vi "OCP.vi"(3 "Data In":dbl[][](array[numeric]), 4 "Timing":T7={"Resolution (ms)"=0.0, "index"=0, "Duty cycle array size"=0, "Pre-scan rest (ms)"=2000}, 9 "Arduino In":cluster{"error in":errorcluster, "LINX  in":T1}) -> (0 "Data Out":dbl[][](array[numeric]), 1 "Aquisition":T8, 2 "Stop condition":bool, 6 "Arduino Out":cluster{"error out":errorcluster, "LINX out":T1})   [LabVIEW 2022 SP3]
uses:
  <vilib>/MakerHub/LINX/Private/Type Defs/LINX Ref.ctl
  <vilib>/MakerHub/LINX/Private/Type Defs/Platform.ctl
  <vilib>/MakerHub/LINX/Private/Type Defs/Interface.ctl
  <vilib>/MakerHub/LINX/Private/Device/Type Defs/LINX Device Config.ctl
  <vilib>/MakerHub/LINX/Private/Device/Type Defs/TCP Config.ctl
  <vilib>/MakerHub/LINX/Private/Device/Type Defs/Channels.ctl
  <vilib>/MakerHub/LINX/Public/Peripherals/Analog/Analog Read 1 Chan.vi
  <vilib>/MakerHub/LINX/Public/Peripherals/Analog/Analog Read N Chans.vi
  <vilib>/MakerHub/LINX/Private/Local IO/LinxAnalogRead.vi
  <vilib>/MakerHub/LINX/Public/Utilities/Check Channel.vi
  <vilib>/MakerHub/LINX/Private/Utilties/Generate Error.vi
  <vilib>/MakerHub/LINX/LMH-LINX.lvlib
  <vilib>/MakerHub/LINX/Private/Device/Device.lvlib
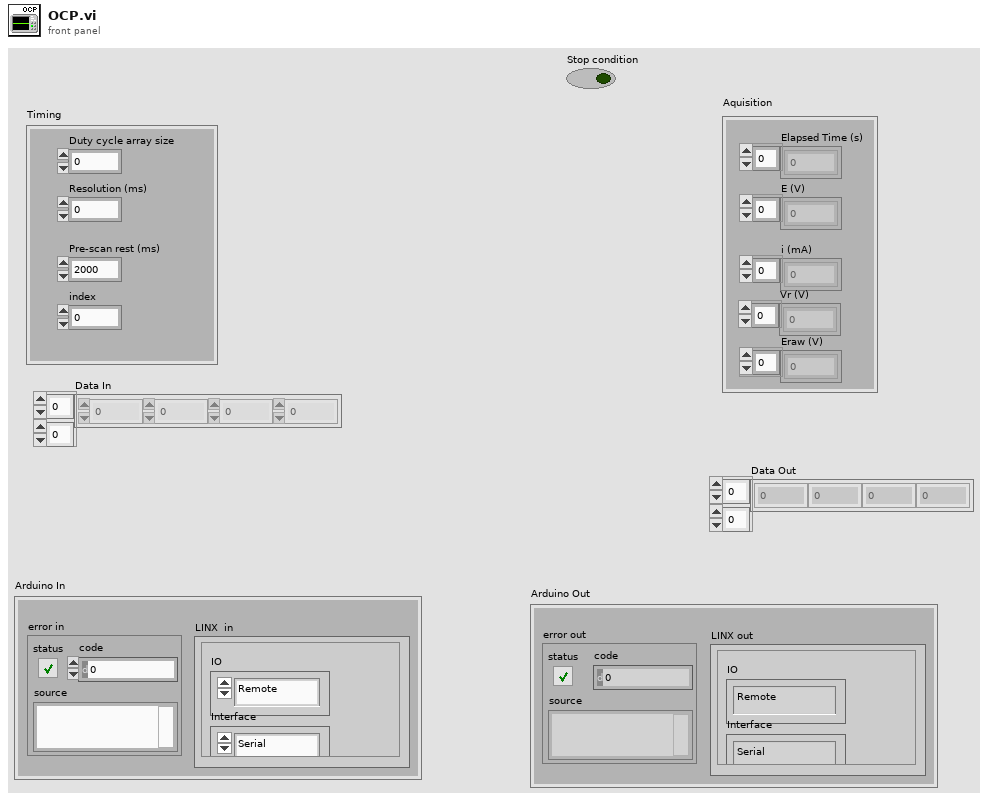
[diagram p1: front panel]
types:
  T1 = typedef "LMH-LINX.lvlib/LINX Ref.ctl" = cluster{"IO":T2, "Interface":T3, "LINX Device Config":T4}
  T2 = typedef "LMH-LINX.lvlib/Platform.ctl" = enum16{"Remote", "Local"}
  T3 = typedef "LMH-LINX.lvlib/Interface.ctl" = enum16{"Serial", "TCP"}
  T4 = typedef "LMH-LINX.lvlib/Device.lvlib/LINX Device Config.ctl" = cluster{"Interface":T3, "COM Port":refnum<visa-resource-name>, "TCP Configuration":T5, "Device Family":u8, "Device ID":u8, "Device Name":string, "TCP Ref":refnum<k5>, "Channels":T6}
  T5 = typedef "LMH-LINX.lvlib/Device.lvlib/TCP Config.ctl" = cluster{"IP Address":string, "Port":u16}
  T6 = typedef "LMH-LINX.lvlib/Channels.ctl" = cluster{"DI":u8[], "DO":u8[], "AI":u8[], "AO":u8[], "PWM":u8[], "QE":u8[], "UART":u8[], "I2C 2":u8[], "SPI":u8[], "CAN":u8[], "Servo":u8[], "AI Ref (V)":dbl, "AI Resolution (Bits)":u8, "AO Ref (V)":dbl, "AO Resolution (Bits)":u8}
  T7 = cluster{"Resolution (ms)":dbl, "index":i32, "Duty cycle array size":i32, "Pre-scan rest (ms)":u32}
  T8 = cluster{"Elapsed Time (s)":dbl[], "E (V)":dbl[], "i (mA)":dbl[], "Vr (V)":dbl[], "Eraw (V)":dbl[]}
  T9 = cluster{"Error Out":errorcluster, "LINX Resource":T1}
  T10 = cluster{dbl[], dbl[], "subarray":dbl[], "subarray":dbl[], "subarray":dbl[]}
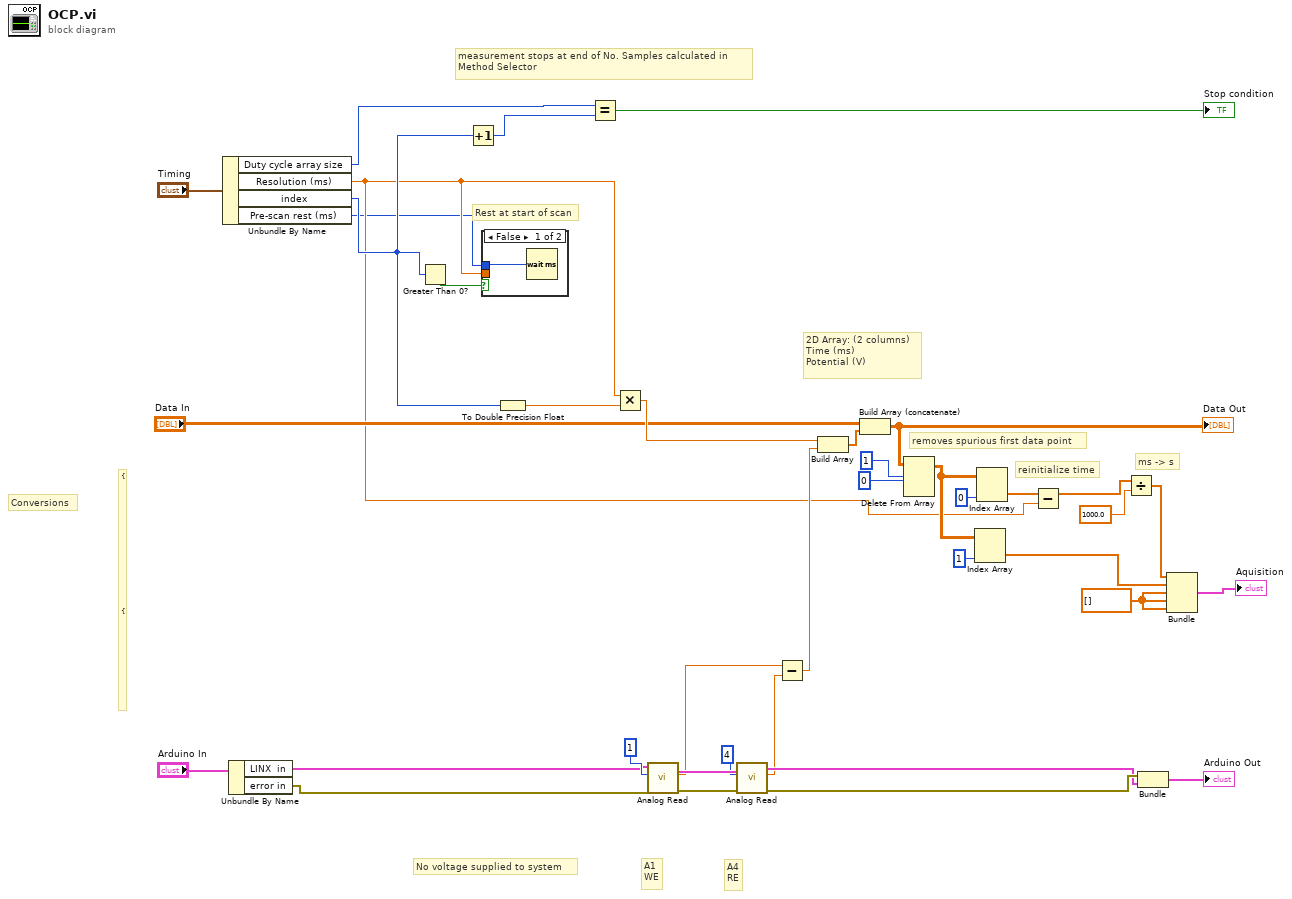
[diagram p0: block diagram]
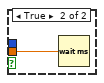
[diagram p2: hidden frame]
diagram:
  w1 = dbl[] [] ("subarray")
  # "Rest at start of scan"
  # "reinitialize time"
  # "ms -> s"
  # "removes spurious first data point"
  # "2D Array: (2 columns)\nTime (ms)\nPotential (V)"
  # "Conversions"
  # "{\n\n\n\n\n\n\n\n\n\n\n\n\n\n\n{"
  # "measurement stops at end of No. Samples calculated in\nMethod Selector"
  # "No voltage supplied to system"
  # "A1\nWE"
  # "A4\nRE"
  n1 = Unbundle By Name("Timing") -> ("Duty cycle array size"=w21:i32, "Resolution (ms)"=w5:dbl, "index"=w6:i32, "Pre-scan rest (ms)"=w4:u32)
  n2 = Unbundle By Name("Arduino In") -> ("LINX  in"=w19:T1, "error in"=w18:errorcluster)
  n3 = Greater Than 0?(x=w6) -> (x > 0?=w7:bool)
  n4 = Increment(x=w6) -> (x+1=w33:i32)
  n5 = case shown="False" w7 {
    tunnel: w5 -> [_ w40]
    tunnel: w4 -> [w39 _]
    frame False {
      n6 = Wait (ms)(milliseconds to wait=w39) -> ()  [unwired: 1 out]
    }
    frame True {
      n7 = Wait (ms)(milliseconds to wait=w40) -> ()  [unwired: 1 out]
    }
  }
  n8 = To Double Precision Float(number=w6) -> (double precision float=w3:dbl)
  n9 = Equal?(x=w21, y=w33) -> (x = y?=→"Stop condition":bool)
  n10 = Multiply(x=w5, y=w3) -> (x*y=w32:dbl)
  n11 = call-poly <vilib>:"Analog Read.vi"("Error In"=w18, "Analog Channel"=u8 1, "LINX Resource"=w19) -> ("Error Out"=w37:errorcluster, "Voltage"=w11:dbl, "LINX Resource"=w36:T1)  [unwired: 5 in, 1 out]
  n12 = call-poly <vilib>:"Analog Read.vi"("Error In"=w37, "Analog Channel"=u8 4, "LINX Resource"=w36) -> ("Error Out"=w16:errorcluster, "Voltage"=w10:dbl, "LINX Resource"=w15:T1)  [unwired: 5 in, 1 out]
  n13 = Subtract(x=w11, y=w10) -> (x-y=w9:dbl)
  n14 = Build Array(w32, w9) -> (w31:dbl[])
  n15 = Build Array (concatenate)("Data In", w31) -> (w12:dbl[][])
  "Data Out" <- w12
  n16 = Delete From Array(array=w12, length=1, index (row)=0) -> (array with subset deleted=w24:dbl[][])  [unwired: 1 in, 1 out]
  n17 = Index Array(array=w24, index (col)=1 ("disabled index (col)")) -> (element=w22:dbl[])  [unwired: 1 in]
  n18 = Index Array(array=w24, index (col)=0 ("disabled index (col)")) -> (element=w27:dbl[])  [unwired: 1 in]
  n19 = Subtract(x=w27, y=w5) -> (x-y=w14:dbl[])
  n20 = Divide(x=w14, y=1000.0) -> (x/y=w23:dbl[])
  n21 = Bundle("Error Out"=w16, "LINX Resource"=w15) -> (→"Arduino Out":T9)  [unwired: 1 in]
  n22 = Bundle(w23, w22, "subarray"=w1, "subarray"=w1, "subarray"=w1) -> (→"Aquisition":T10)  [unwired: 1 in]
